vi "FitGaussian.vi"(0 "X":sgl[](array[numeric]), 5 "Y":sgl[](array[numeric]), 7 "Amplitude fit":dbl=1000.0, 9 "Initial X":dbl=800.0, 11 "FWHM":dbl=10.0, 12 "Offset":dbl=1000.0, 13 "tolerance":dbl=1e-05 format="%#_3g") -> (4 "Fit Spectrum":cluster{sgl[], "Best Gaussian Fit":dbl[]}(graph), 6 "amplitude":dbl, 8 "center":dbl, 10 "standard deviation":dbl, 15 "FWHM":dbl)   [LabVIEW 2012]
uses:
  <vilib>/Analysis/NI_AALPro.lvlib
panel:
  out "residue":dbl
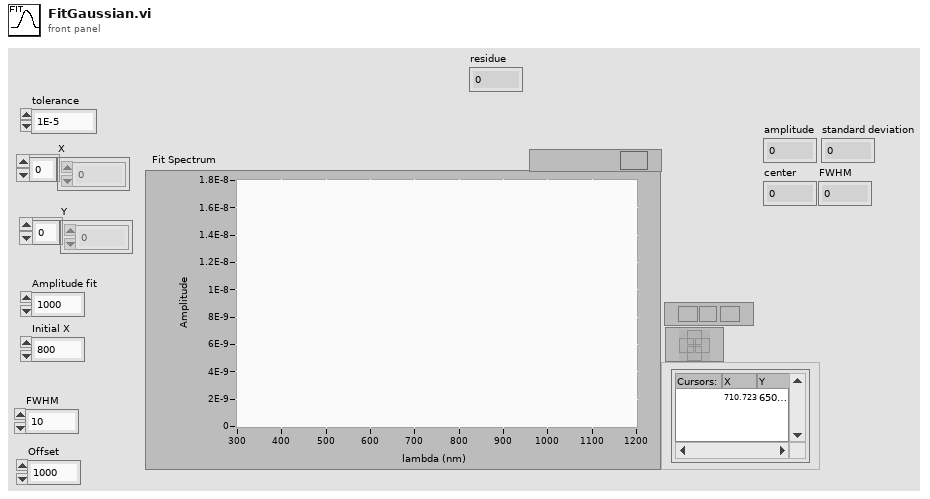
[diagram p1: front panel]
types:
  T1 = cluster{"amp min":dbl, "amp max":dbl, "center min":dbl, "center max":dbl, "deviation min":dbl, "deviation max":dbl, "offset min":dbl, "offset max":dbl}
  T2 = cluster{"Amplitude fit":dbl, "Initial X":dbl, dbl, "Offset":dbl}
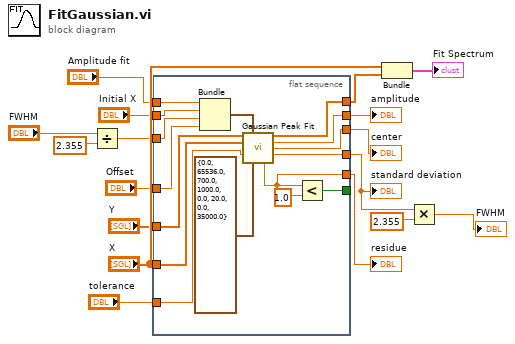
[diagram p0: block diagram]
diagram:
  n1 = Divide(x="FWHM", y=2.355) -> (x/y=w2:dbl)
  n2 = flat-sequence {
    tunnel: "X" -> [w33]
    tunnel: "Y" -> [w32]
    tunnel: [w31] -> w14
    tunnel: [w30] -> w13
    tunnel: [w29] -> w12
    tunnel: [w28] -> w11
    tunnel: "tolerance" -> [w27]
    tunnel: [w26] -> w5
    tunnel: [w24] -> _
    tunnel: "Amplitude fit" -> [w23]
    tunnel: "Initial X" -> [w22]
    tunnel: w2 -> [w21]
    tunnel: "Offset" -> [w20]
    frame #0 {
      n3 = Bundle("Amplitude fit"=w23, "Initial X"=w22, w21, "Offset"=w20) -> (w19:T2)  [unwired: 1 in]
      n4 = call <vilib>:"Gaussian Peak Fit.vi"("Y"=w32, "initial guess"=w19, "X"=w33, "tolerance"=w27, "parameter bounds"=T1 {"amp min"=0.0, "amp max"=65536.0, "center min"=700.0, "center max"=1000.0, "deviation min"=0.0, "deviation max"=20.0, "offset min"=0.0, "offset max"=35000.0}) -> ("Best Gaussian Fit"=w31:dbl[], "amplitude"=w30:dbl, "center"=w29:dbl, "standard deviation"=w28:dbl, "residue"=w26:dbl)  [unwired: 4 in, 2 out]
      n5 = Less?(x=w26, y=1.0) -> (x < y?=w24:bool)
    }
  }
  n6 = Bundle("X"="X", "Best Gaussian Fit"=w14) -> (→"Fit Spectrum":cluster{"X":sgl[], "Best Gaussian Fit":dbl[]})  [unwired: 1 in]
  n7 = Multiply(x=w11, y=2.355) -> (x*y=→"FWHM":dbl)
  "amplitude" <- w13
  "center" <- w12
  "standard deviation" <- w11
  "residue" <- w5
